vi "DSDLL Initialize.vi"(8 "error in":errorcluster, 11 "dsdll session":T1) -> (0 "error out":errorcluster, 3 "dsdll session out":T1)   [LabVIEW 2020, in "DSDLL Virtual Digitizer.lvlib"]
doc: "Initializes DSDLL lib. Must becalled before any other funcion can be used (just once)."
uses:
  DSDLL Virtual Digitizer.lvlib
  DSDLL Session.ctl
  dsdll/dsdll_instance.ctl
  dsdll/dsdll_device_record.ctl
  DSDLL Process Config.ctl
  DSDLL Data Packet.ctl
  dsdll/dsdll.lvlib
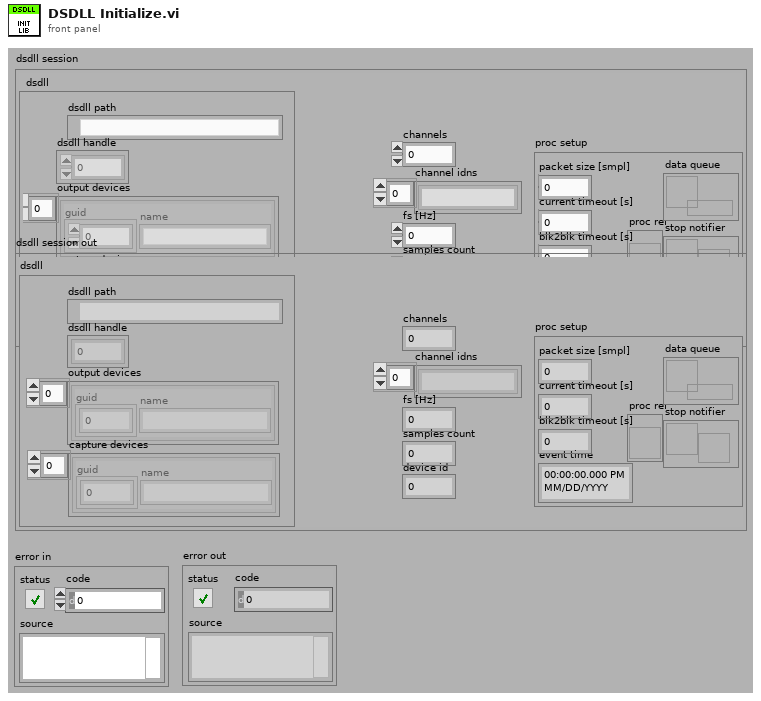
[diagram p1: front panel]
types:
  T1 = typedef "DSDLL Virtual Digitizer.lvlib/DSDLL Session.ctl" = cluster{"dsdll":T2, "channels":i32, "device id":i32, "channel idns":string[], "proc setup":T4, "samples count":i32, "fs [Hz]":dbl}
  T2 = typedef "dsdll.lvlib/dsdll_instance.ctl" = cluster{"dsdll path":path, "dsdll handle":u8[], "output devices":T3[], "capture devices":T3[]}
  T3 = typedef "dsdll.lvlib/dsdll_device_record.ctl" = cluster{"guid":u8[], "name":string}
  T4 = typedef "DSDLL Virtual Digitizer.lvlib/DSDLL Process Config.ctl" = cluster{"packet size [smpl]":i32, "current timeout [s]":dbl, "blk2blk timeout [s]":dbl, "event time":timestamp, "data queue":refnum<queue>, "stop notifier":refnum<notifier>, "proc ref":refnum<vi>}
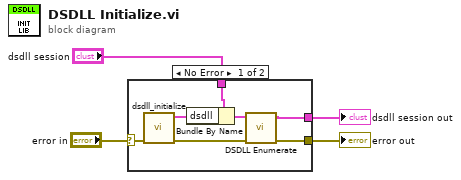
[diagram p0: block diagram]
diagram:
  n1 = case shown="No Error" "error in" {
    selector: "error in" -> [w5 w13]
    tunnel: [w10 w13] -> w4
    tunnel: "dsdll session" -> [w8 w12]
    tunnel: [w6 w12] -> w2
    frame No Error {
      n2 = call "dsdll_initialize.vi"("error in"=w5) -> ("error out"=w11:errorcluster, "dsdll instance out"=w9:T2)  [unwired: 9 in]
      n3 = Bundle By Name(cluster=w8, "dsdll"=w9) -> (w7:T1)
      n4 = call "DSDLL Enumerate.vi"("error in"=w11, "dsdll session"=w7) -> ("error out"=w10:errorcluster, "dsdll session out"=w6:T1)  [unwired: 7 in, 1 out]
    }
    frame Error {
    }
  }
  "error out" <- w4
  "dsdll session out" <- w2
